vi "Read Measurement (Signal Point).vi"(0 "VISA resource name":refnum<visa-resource-name>, 5 "Time Value (0 S)":dbl, 11 "error in (no error)":errorcluster) -> (4 "VISA resource name out":refnum<visa-resource-name>, 6 "Vertical Value":dbl, 15 "error out":errorcluster)   [LabVIEW 2017, in "Agilent 2000 3000 X-Series.lvlib"]
doc: "Returns the value at a specified time on the source."
uses:
  Agilent 2000 3000 X-Series.lvlib
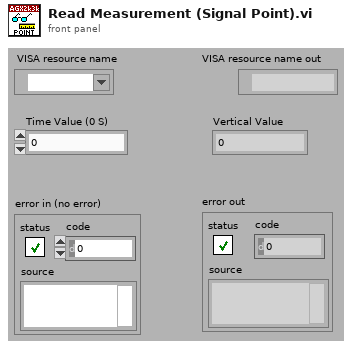
[diagram p1: front panel]
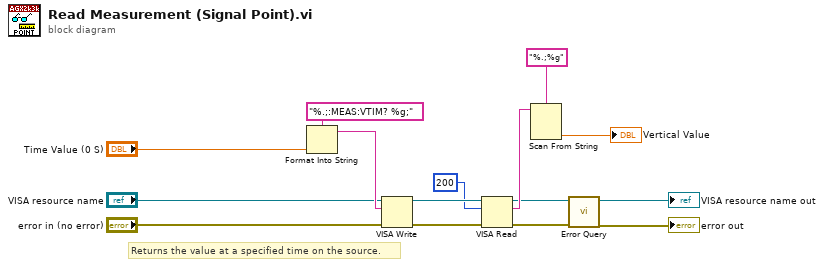
[diagram p0: block diagram]
diagram:
  # "Returns the value at a specified time on the source."
  n1 = Format Into String(format string="%.;:MEAS:VTIM? %g;", "Time Value (0 S)") -> (resulting string=w13:string)  [unwired: 2 in, 1 out]
  n2 = VISA Write(VISA resource name="VISA resource name", write buffer=w13, error in (no error)="error in (no error)") -> (VISA resource name out=w7:refnum<visa-resource-name>, error out=w6:errorcluster)  [unwired: 1 out]
  n3 = VISA Read(VISA resource name=w7, byte count=u32 200, error in (no error)=w6) -> (VISA resource name out=w5:refnum<visa-resource-name>, read buffer=w8:string, error out=w4:errorcluster)  [unwired: 1 out]
  n4 = Scan From String(format string="%.;%g", input string=w8) -> (output 1=→"Vertical Value":dbl)  [unwired: 2 in, 4 out]
  n5 = call "Error Query.vi"("error in (no error)"=w4, "VISA resource name"=w5) -> ("error out"=→"error out":errorcluster, "VISA resource name out"=→"VISA resource name out":refnum<visa-resource-name>)  [unwired: 8 out]
